vi "Helicopter - Draw Model.vi"(6 "error in":errorcluster, 7 "Reset?":bool, 8 "Pitch":dbl, 9 "Travel":dbl, 10 "Elevation":dbl, 11 "Path to 3D model":path) -> (0 "error out":errorcluster, 3 "Scene.New Object":refnum<vi>)   [LabVIEW 2013]
doc: "This VI draws the Flexible Joint using the \"LabVIEW 3D Picture Control Evaluation Software\".\nThe evaluation software can be downloaded from the following URL: http://digital.ni.com/express.nsf/express?openagent&code=exn4gy"
uses:
  <vilib>/picture/3D Picture Control/NI_3D Picture Control.lvlib
panel:
  out "3D Picture Control":refnum<vi>(3d-picture)
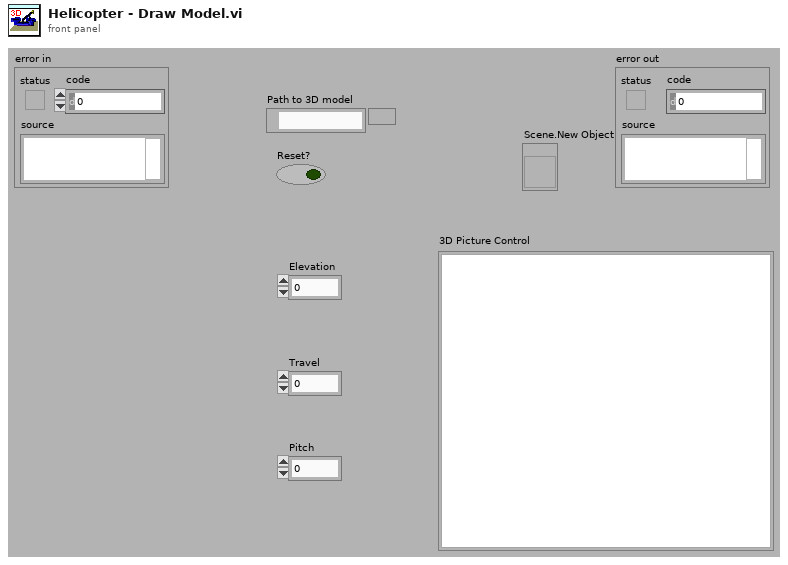
[diagram p1: front panel]
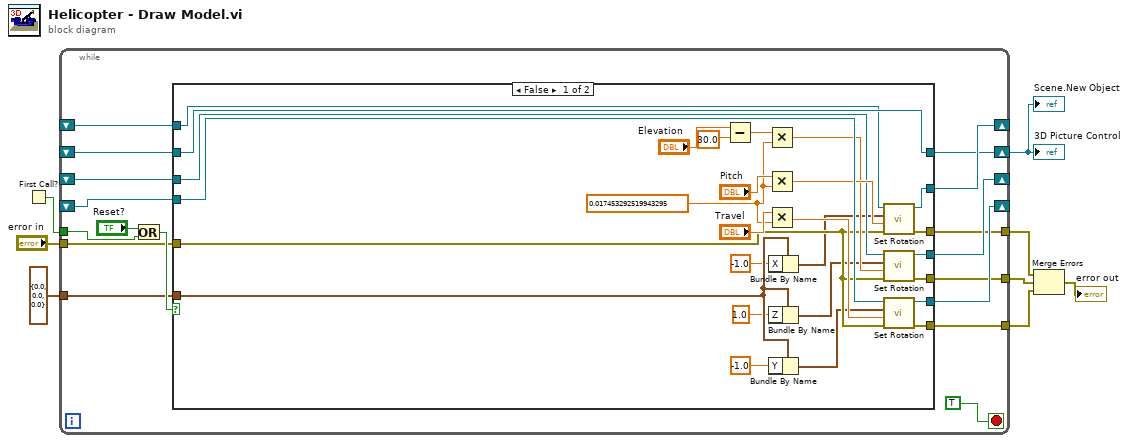
[diagram p0: block diagram]
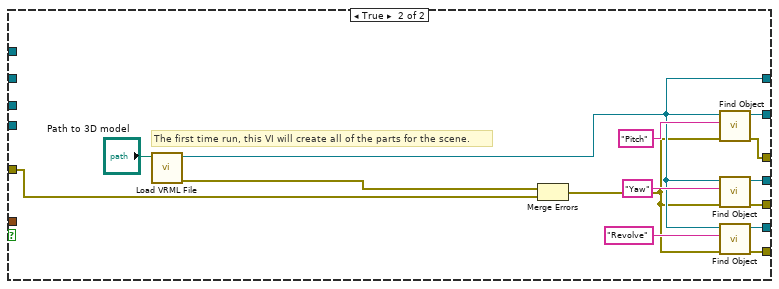
[diagram p2: hidden frame]
diagram:
  n1 = First Call?() -> (First Call?: T/F=w8:bool)
  n2 = while {
    shift-right: [w17] -> w7
    shift-left: _ -> [w16]
    shift-right: [w24] -> _
    shift-left: _ -> [w23]
    shift-right: [w22] -> _
    shift-left: _ -> [w21]
    tunnel: w8 -> [w18]
    shift-right: [w15] -> _
    shift-left: _ -> [w14]
    tunnel: "error in" -> [w12]
    tunnel: [w13] -> w5
    tunnel: [w11] -> w4
    tunnel: [w10] -> w3
    tunnel: cluster{"X":sgl, "Y":sgl, "Z":sgl} {"X"=0.0, "Y"=0.0, "Z"=0.0} ("Axis") -> [w9]
    stop <- TRUE stop-if-true
    n3 = Or(x="Reset?", y=w18) -> (x .or. y?=w20:bool)
    n4 = case shown="False" w20 {
      tunnel: [w44 w63] -> w24
      tunnel: w23 -> [w46 _]
      tunnel: [w42 w64] -> w22
      tunnel: w21 -> [w43 _]
      tunnel: [w47 w61] -> w17
      tunnel: w16 -> [w47 _]
      tunnel: [w39 w60] -> w15
      tunnel: w14 -> [w38 _]
      tunnel: [w36 w58] -> w13
      tunnel: w12 -> [w35 w55]
      tunnel: [w34 w57] -> w11
      tunnel: [w33 w56] -> w10
      tunnel: w9 -> [w32 _]
      frame False {
        w37 = 0.017453292519943295 ("x/y")
        n5 = Subtract(x="Elevation", y=30.0) -> (x-y=w49:dbl)
        n6 = Multiply(x=w49, y=w37) -> (x*y=w40:dbl)
        n7 = Multiply(x="Pitch", y=w37) -> (x*y=w41:dbl)
        n8 = Multiply(x="Travel", y=w37) -> (x*y=w45:dbl)
        n9 = Bundle By Name(cluster=w32, "X"=sgl -1.0) -> (w28:cluster{"X":sgl, "Y":sgl, "Z":sgl})
        n10 = Bundle By Name(cluster=w32, "Z"=sgl 1.0) -> (w29:cluster{"X":sgl, "Y":sgl, "Z":sgl})
        n11 = Bundle By Name(cluster=w32, "Y"=sgl -1.0) -> (w27:cluster{"X":sgl, "Y":sgl, "Z":sgl})
        n12 = call <vilib>:"Set Rotation.vi"("error in (no error)"=w35, "Angle"=w41, "Axis"=w28, "Scene Object"=w43) -> ("error out"=w36:errorcluster, "Rotated Scene Object"=w42:refnum<vi>)  [unwired: 6 out]
        n13 = call <vilib>:"Set Rotation.vi"("error in (no error)"=w35, "Angle"=w40, "Axis"=w29, "Scene Object"=w38) -> ("error out"=w34:errorcluster, "Rotated Scene Object"=w39:refnum<vi>)  [unwired: 6 out]
        n14 = call <vilib>:"Set Rotation.vi"("error in (no error)"=w35, "Angle"=w45, "Axis"=w27, "Scene Object"=w46) -> ("error out"=w33:errorcluster, "Rotated Scene Object"=w44:refnum<vi>)  [unwired: 6 out]
      }
      frame True {
        # "The first time run, this VI will create all of the parts for the scene."
        n15 = call <vilib>:"Load VRML File.vi"("Path"="Path to 3D model") -> ("error out"=w54:errorcluster, "Scene:Read Scene File"=w61:refnum<vi>)  [unwired: 1 in, 8 out]
        n16 = Merge Errors(w54, w55) -> (w53:errorcluster)
        n17 = call <vilib>:"Find Object.vi"("error in (no error)"=w53, "Object Name"="Pitch" ("Name"), "Scene Refnum"=w61) -> ("error out"=w58:errorcluster, "Object Refnum"=w64:refnum<vi>)  [unwired: 7 out]
        n18 = call <vilib>:"Find Object.vi"("error in (no error)"=w53, "Object Name"="Yaw" ("Name"), "Scene Refnum"=w61) -> ("error out"=w57:errorcluster, "Object Refnum"=w60:refnum<vi>)  [unwired: 7 out]
        n19 = call <vilib>:"Find Object.vi"("error in (no error)"=w53, "Object Name"="Revolve" ("Name"), "Scene Refnum"=w61) -> ("error out"=w56:errorcluster, "Object Refnum"=w63:refnum<vi>)  [unwired: 7 out]
      }
    }
  }
  "Scene.New Object" <- w7
  "3D Picture Control" <- w7
  n20 = Merge Errors(w5, w4, w3) -> (→"error out":errorcluster)
